vi "generate table.vi"(7 "table":T1, 8 "error in":errorcluster, 10 "engine configuration":refnum<class "engine configuration.lvclass">, 11 "tag bus configurable plugin module configuration":refnum<class "io configuration.lvclass">) -> (0 "error out":errorcluster)   [LabVIEW 2014, in "io editor node.lvclass"]
uses:
  io editor node.lvclass
  table reference.ctl
  <vilib>/NI/Module Execution Interface/Engine Configuration/engine configuration.lvclass
  configuration/io configuration.lvclass
  <vilib>/NI/Configuration Framework/serializable configuration/NISE_CEF_serializable configuration.lvclass/NISE_CEF_serializable configuration.ctl
  table line.ctl
  <vilib>/NI/Tag Bus Module Framework/channel/TBM channel.lvclass
  <vilib>/NI/Tag Bus/tag/tag descriptor.lvclass/tag descriptor.ctl
  <vilib>/NI/Tag Bus/tag/read tag name.vi
  <vilib>/NI/Configuration Framework/serializable configuration/Read UID.vi
  <vilib>/Utility/LVClass/Get LV Class Name.vi
  <vilib>/NI/Configuration Framework/error generator/NISE_error generator.vi
  <vilib>/NI/Tag Bus/tag/tag descriptor.lvclass
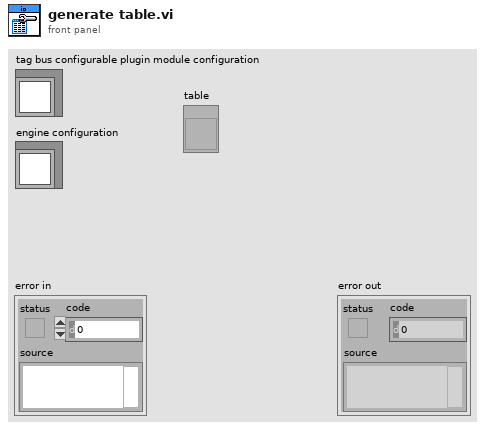
[diagram p1: front panel]
types:
  T1 = typedef "io editor node.lvclass/table reference.ctl" = refnum<vi>
  T2 = typedef "io editor node.lvclass/table line.ctl" = cluster{"channel":refnum<class "TBM channel.lvclass">, "tag name":string}
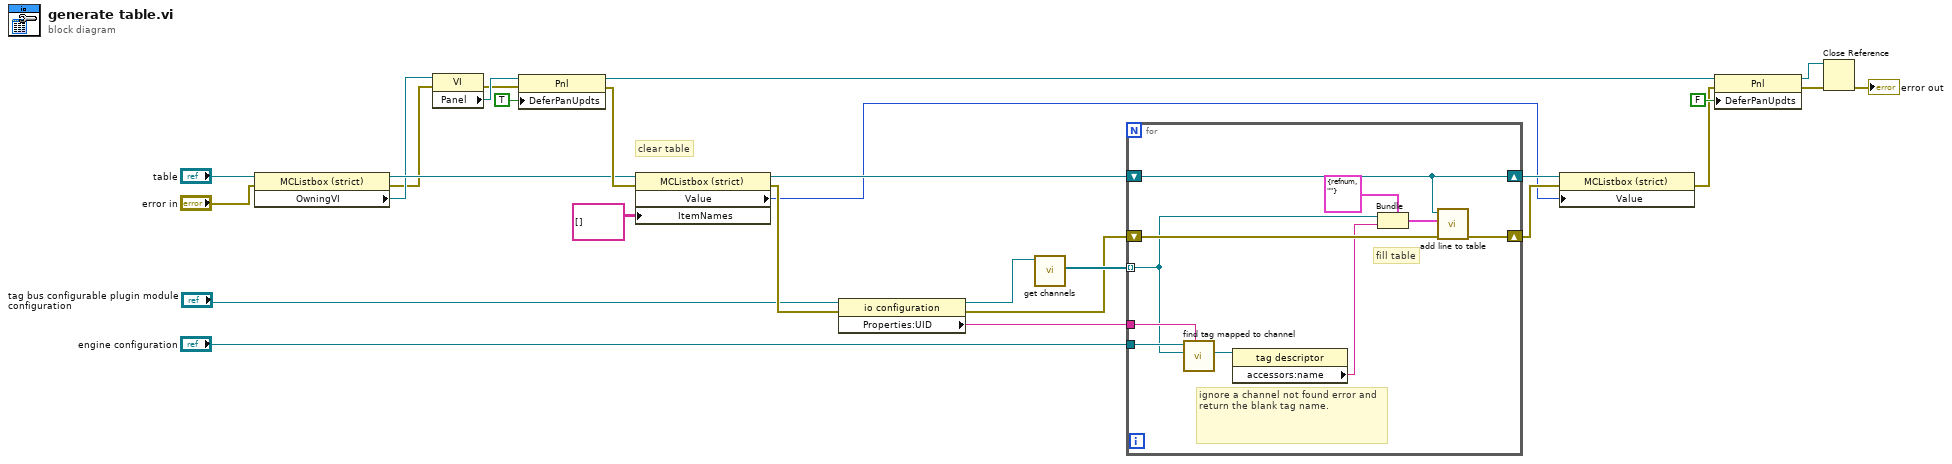
[diagram p0: block diagram]
diagram:
  # "clear table"
  n1 = property class="MCListbox (strict)"(reference="table", error in="error in") -> (reference out=w7:T1, error out=w4:errorcluster, "OwningVI"=w5:refnum<vi>)
  n2 = property class="VI"(reference=w5, error in=w4) -> (error out=w13:errorcluster, "Panel"=w14:refnum<vi>)  [unwired: 1 out]
  n3 = property class="Pnl"(reference=w14, error in=w13, "DeferPanUpdts"=TRUE ("Defer Panel Updates")) -> (reference out=w10:refnum<vi>, error out=w12:errorcluster)
  n4 = property class="MCListbox (strict)"(reference=w7, error in=w12, "ItemNames"=string[][] [] ("Item Names")) -> (reference out=w25:T1, error out=w21:errorcluster, "Value"=w16:i32)
  n5 = property class="io configuration"(reference="tag bus configurable plugin module configuration", error in=w21) -> (reference out=w23:refnum<class "io configuration.lvclass">, error out=w20:errorcluster, "Properties:UID"=w22:string)
  n6 = call-dynamic "get channels.vi"("io configuration in"=w23) -> ("channels"=w26:refnum<class "TBM channel.lvclass">[])  [unwired: 9 in, 1 out]
  n7 = for {
    shift-right: [w37] -> w17
    shift-left: w20 -> [w34]
    tunnel: w26 -> [w31] mode=indexing
    tunnel: "engine configuration" -> [w33]
    tunnel: w22 -> [w32]
    shift-right: [w28] -> w18
    shift-left: w25 -> [w28]
    # "ignore a channel not found error and return the blank tag name."
    # "fill table"
    n8 = call <vilib>:"find tag mapped to channel.vi"("owner"=w32, "channel"=w31, "engine configuration in"=w33) -> ("tag"=w30:refnum<class "tag descriptor.lvclass">)  [unwired: 6 in, 2 out]
    n9 = property class="tag descriptor"(reference=w30) -> ("accessors:name"=w29:string)  [unwired: 1 in, 2 out]
    n10 = Bundle(cluster=T2 {"channel"=refnum, "tag name"=""} ("line"), "channel"=w31, "tag name"=w29) -> (w35:T2)
    n11 = call "add line to table.vi"("error in"=w34, "line"=w35, "operations table"=w28) -> ("error out"=w37:errorcluster)  [unwired: 8 in]
  }
  n12 = property class="MCListbox (strict)"(reference=w18, error in=w17, "Value"=w16) -> (error out=w9:errorcluster)  [unwired: 1 out]
  n13 = property class="Pnl"(reference=w10, error in=w9, "DeferPanUpdts"=FALSE ("Defer Panel Updates")) -> (reference out=w2:refnum<vi>, error out=w8:errorcluster)
  n14 = Close Reference(reference=w2, error in (no error)=w8) -> (error out=→"error out":errorcluster)
